vi "Async Get averaged image from CamServer.vi"(0 "Image directory path":path=path "C:/test", 1 "Image name":string="test", 2 "Duration (s)":dbl=10.0 format="%#_13g", 3 "Averaging time (s) (from end)":dbl=1.0 format="%#_13g", 4 "Camera":T1="Travcam") -> (5 "Image file path":path, 6 "Error out":errorcluster)   [LabVIEW 2015]
doc: "Asynchronously gets a time-averaged image from the selected camera on the camera server and saves it to the specified path with specified name.s"
uses:
  Camera enum/Camera enum.ctl
  Globals/CamServer global.vi
panel:
  # "PN 21/08/15"
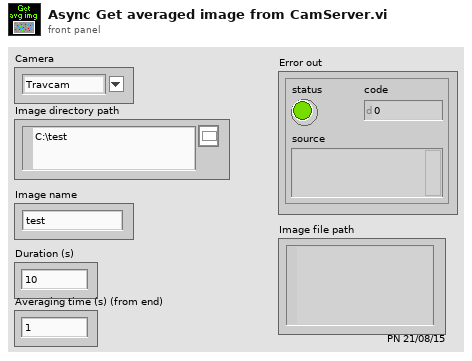
[diagram p1: front panel]
types:
  T1 = typedef "Camera enum.ctl" = string
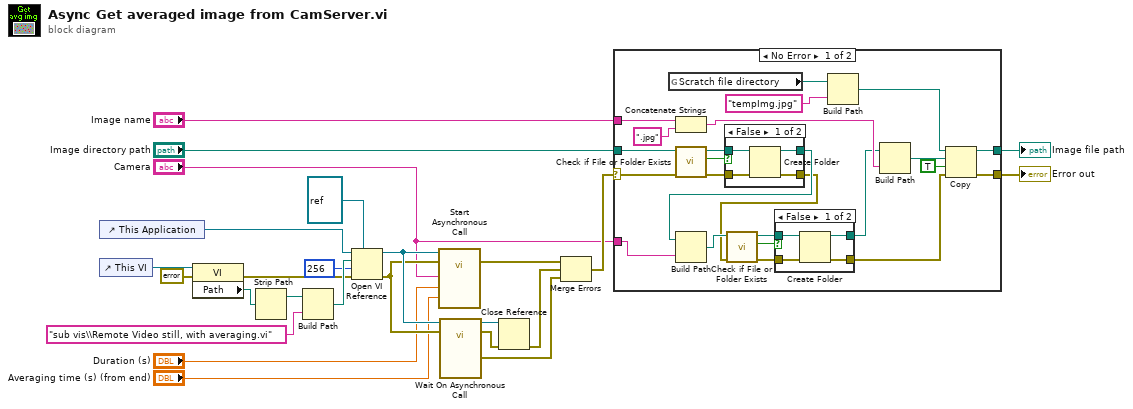
[diagram p0: block diagram]
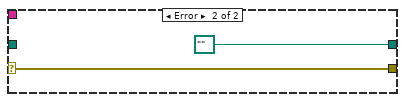
[diagram p4: hidden frame]
diagram:
  n1 = control-ref of="This Application"() -> (w20:refnum<vi>)
  n2 = control-ref of="This VI"() -> (w25:refnum<vi>)
  n3 = property class="VI"(reference=w25, error in=errorcluster {"status"=FALSE, "code"=0, "source"=""} ("error in (no error)")) -> (error out=w22:errorcluster, "Path"=w18:path)  [unwired: 1 out]
  n4 = Strip Path(path=w18) -> (stripped path=w17:path)  [unwired: 1 out]
  n5 = Build Path(base path=w17, name or relative path="sub vis\\Remote Video still, with averaging.vi") -> (appended path=w23:path)
  n6 = Open VI Reference(type specifier VI Refnum (for type only)=refnum<vi> refnum, application reference (local)=w20, vi path=w23, options=256, error in (no error)=w22) -> (vi reference=w16:refnum<vi>, error out=w15:errorcluster)  [unwired: 1 in]
  n7 = call-by-ref "Start Asynchronous Call"(reference=w16, error in=w15, "Averaging time (s) (from end)"="Averaging time (s) (from end)", "Duration (s)"="Duration (s)", "Camera"="Camera") -> (error out=w13:errorcluster)  [unwired: 2 out]
  n8 = call-by-ref "Wait On Asynchronous Call"(reference=w16, error in=w15) -> (reference out=w14:refnum<vi>, error out=w12:errorcluster, "Error out"=w10:errorcluster)  [unwired: 3 in]
  n9 = Close Reference(reference=w14, error in (no error)=w12) -> (error out=w11:errorcluster)
  n10 = Merge Errors(w13, w11, w10) -> (w3:errorcluster)
  n11 = case shown="No Error" w3 {
    selector: w3 -> [w48 w63]
    tunnel: "Image directory path" -> [w49 _]
    tunnel: "Image name" -> [w43 _]
    tunnel: [w27 w63] -> w6
    tunnel: "Camera" -> [w32 _]
    tunnel: [w26 path "" ("new path")] -> w1
    frame No Error {
      n12 = global read "CamServer global.vi" "Scratch file directory"() -> (w38:path)
      n13 = Concatenate Strings(w43, ".jpg" ("string")) -> (w41:string)
      n14 = call <vilib>:"Check if File or Folder Exists.vi"("error in (no error)"=w48, "path"=w49) -> ("error out"=w45:errorcluster, "file or folder exists?"=w47:bool, "dup path"=w46:path)  [unwired: 7 in]
      n15 = case shown="False" w47 {
        tunnel: w46 -> [w59 w61]
        tunnel: w45 -> [w58 w60]
        tunnel: [w57 w61] -> w33
        tunnel: [w56 w60] -> w30
        frame False {
          n16 = Create Folder(path (use dialog)=w59, error in=w58) -> (created path=w57:path, error out=w56:errorcluster)  [unwired: 1 in, 1 out]
        }
        frame True {
        }
      }
      n17 = Build Path(base path=w33, name or relative path=w32) -> (appended path=w31:path)
      n18 = call <vilib>:"Check if File or Folder Exists.vi"("error in (no error)"=w30, "path"=w31) -> ("error out"=w34:errorcluster, "file or folder exists?"=w35:bool, "dup path"=w36:path)  [unwired: 7 in]
      n19 = case shown="False" w35 {
        tunnel: w36 -> [w53 w55]
        tunnel: w34 -> [w52 w54]
        tunnel: [w51 w55] -> w29
        tunnel: [w50 w54] -> w28
        frame False {
          n20 = Create Folder(path (use dialog)=w53, error in=w52) -> (created path=w51:path, error out=w50:errorcluster)  [unwired: 1 in, 1 out]
        }
        frame True {
        }
      }
      n21 = Build Path(base path=w38, name or relative path="tempImg.jpg") -> (appended path=w37:path)
      n22 = Build Path(base path=w29, name or relative path=w41) -> (appended path=w42:path)
      n23 = Copy(8:w28, 9:TRUE ("overwrite (F)"), 10:w42, 11:w37) -> (0:w27:errorcluster, 3:w26:path)  [unwired: 1 in, 1 out]
    }
    frame Error {
    }
  }
  "Error out" <- w6
  "Image file path" <- w1
